vi "Camera_Widefield_old.vi"() -> ()   [LabVIEW 2014]
doc: "Allows the user to focus the camera on the sample"
uses:
  <vilib>/vision/Image Controls.llb/IMAQ Image.ctl
  <vilib>/userdefined/High Color/IMAQdx.ctl
  Widefield_globals.vi
  <vilib>/vision/NI_Vision_Development_Module.lvlib
  <vilib>/vision/driver/NI_Vision_Acquisition_Software.lvlib
  <resource>/objmgr/imaqdx.rc
panel:
  out "Exposure time (ms)":string
  out "Image Buffer":T1
  out "Waveform Graph":u32[](graph)
  in  "Snap":bool
  in  "Exit Focus Loop":bool
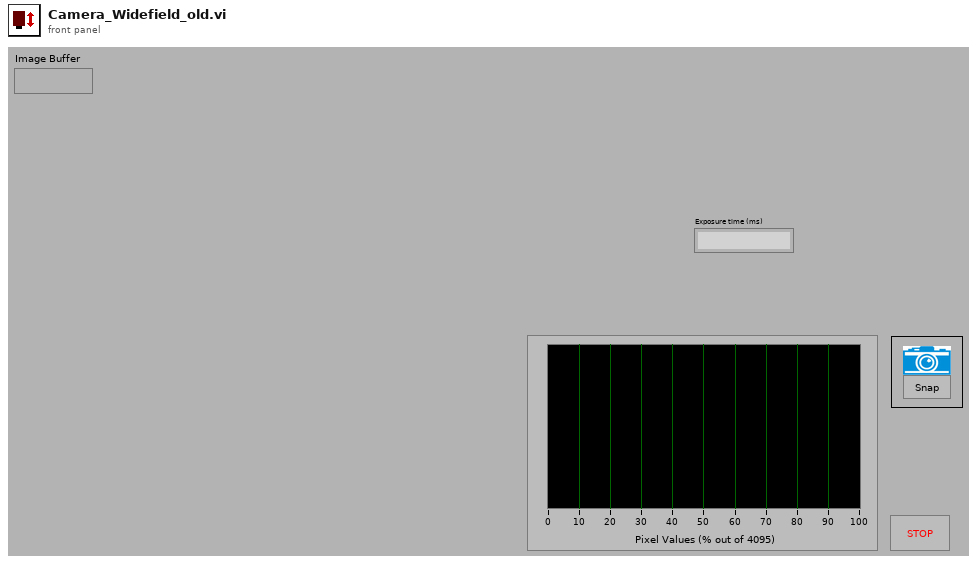
[diagram p1: front panel]
types:
  T1 = typedef "IMAQ Image.ctl" = refnum<image>
  T2 = typedef "IMAQdx.ctl" = refnum<k21>
  T3 = cluster{"histogram":u32[], "Minimal Value":sgl, "Maximal Value":sgl, "Starting Value":sgl, "Interval Width":sgl, "Mean Value":sgl, "Standard  Variation":sgl, "Area (pixels)":i32}
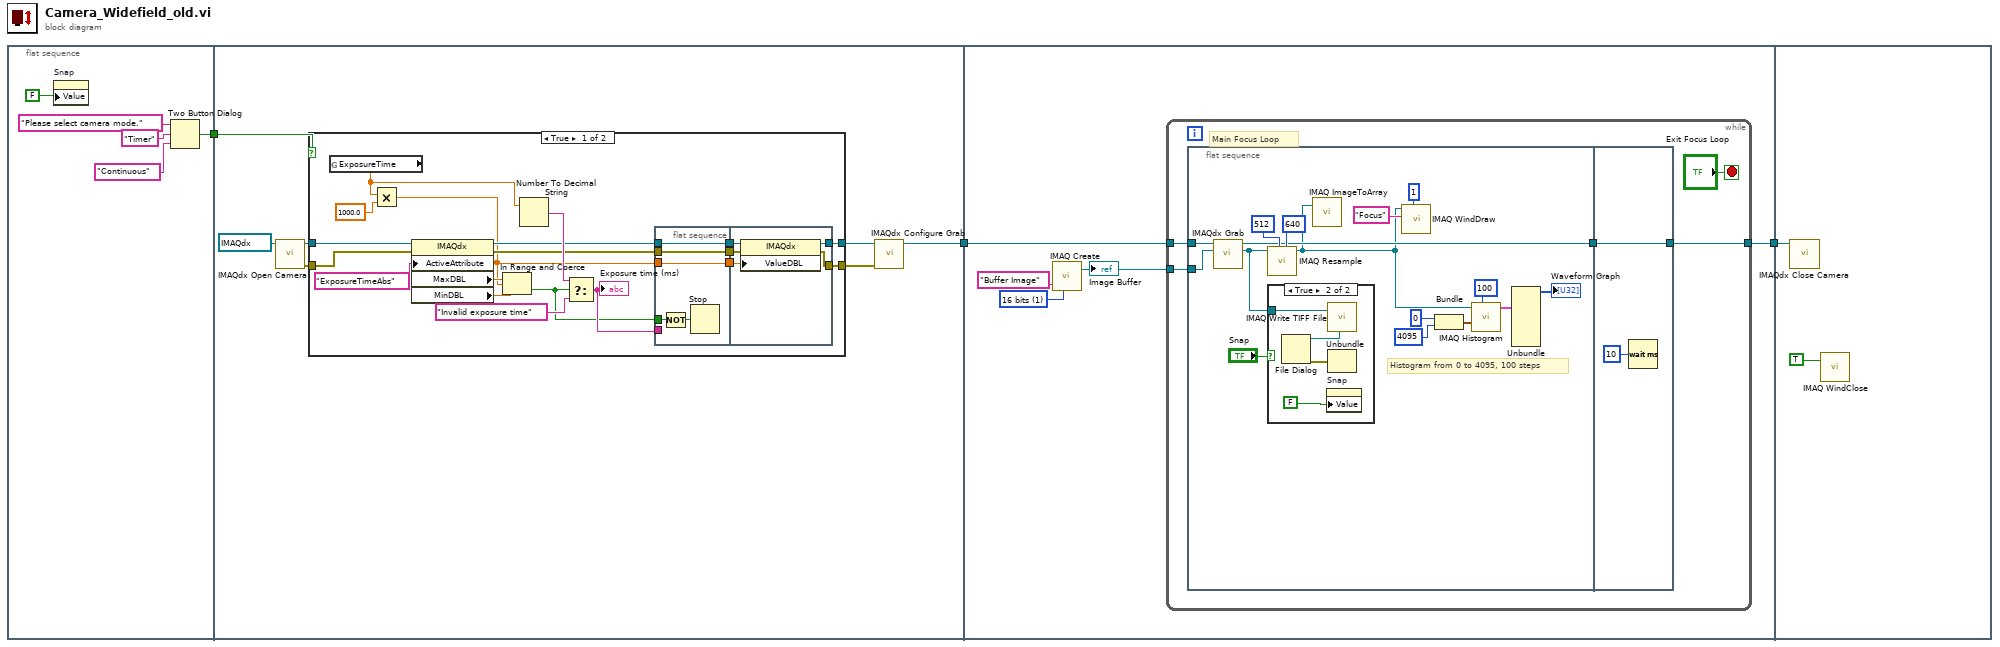
[diagram p0: block diagram]
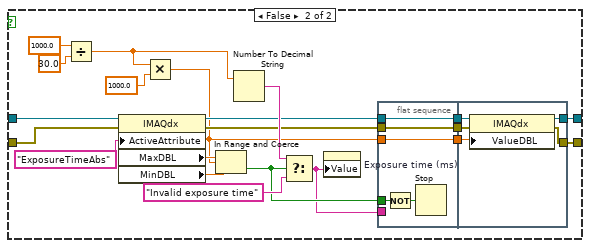
[diagram p2: hidden frame]
diagram:
  n1 = flat-sequence {
    tunnel: [w4] -> w3
    tunnel: w3 -> [w12]
    tunnel: [w9] -> w2
    tunnel: w2 -> [w77]
    tunnel: [w76] -> w1
    tunnel: w1 -> [w108]
    frame #0 {
      n2 = property on="Snap" class="Bool (strict)"("Value"=FALSE ("Snap!")) -> ()  [unwired: 2 in, 2 out]
      n3 = Two Button Dialog(message="Please select camera mode.", 1:"Continuous" ("F button name (\"Cancel\")"), 2:"Timer" ("T button name (\"OK\")")) -> (T button?=w4:bool)
    }
    frame #1 {
      n4 = call <vilib>:"IMAQdx Open Camera.vi"("Session In"=T2 "cam0") -> ("error out"=w13:errorcluster, "Session Out"=w14:T2)  [unwired: 2 in, 7 out]
      n5 = case shown="True" w12 {
        tunnel: [w18 w50] -> w15
        tunnel: w14 -> [w34 w65]
        tunnel: w13 -> [w32 w63]
        tunnel: [w19 w51] -> w10
        frame True {
          n6 = global read "Widefield_globals.vi" "ExposureTime"() -> (w16:dbl)
          n7 = Multiply(x=w16, y=1000.0) -> (x*y=w20:dbl)
          n8 = property class="IMAQdx"(reference=w34, error in=w32, "ActiveAttribute"="ExposureTimeAbs" ("Camera Attribute")) -> (reference out=w25:T2, error out=w24:errorcluster, "MaxDBL"=w31:dbl, "MinDBL"=w17:dbl)
          n9 = In Range and Coerce(upper limit=w31, x=w20, lower limit=w17) -> (In Range?=w26:bool)  [unwired: 1 out]
          n10 = Number To Decimal String(number=w16) -> (decimal integer string=w28:string)  [unwired: 1 out]
          n11 = Select(t=w28, s=w26, f="Invalid exposure time") -> (s? t:f=w27:string)
          "Exposure time (ms)" <- w27
          n12 = flat-sequence {
            tunnel: w27 -> [_]
            tunnel: w26 -> [w38]
            tunnel: w25 -> [w36]
            tunnel: w24 -> [w37]
            tunnel: [w37] -> w23
            tunnel: [w36] -> w22
            tunnel: [w35] -> w21
            tunnel: w20 -> [w35]
            tunnel: w23 -> [w43]
            tunnel: w22 -> [w44]
            tunnel: w21 -> [w42]
            tunnel: [w41] -> w19
            tunnel: [w40] -> w18
            frame #0 {
              n13 = Not(x=w38) -> (.not. x?=w39:bool)
              n14 = Stop(stop? (T)=w39) -> ()
            }
            frame #1 {
              n15 = property class="IMAQdx"(reference=w44, error in=w43, "ValueDBL"=w42) -> (reference out=w41:T2, error out=w40:errorcluster)
            }
          }
        }
        frame False {
          n16 = Divide(x=1000.0 ("y"), y=30.0) -> (x/y=w46:dbl)
          n17 = property class="IMAQdx"(reference=w65, error in=w63, "ActiveAttribute"="ExposureTimeAbs" ("Camera Attribute")) -> (reference out=w57:T2, error out=w56:errorcluster, "MaxDBL"=w62:dbl, "MinDBL"=w49:dbl)
          n18 = Multiply(x=w46, y=1000.0) -> (x*y=w52:dbl)
          n19 = In Range and Coerce(upper limit=w62, x=w52, lower limit=w49) -> (In Range?=w58:bool)  [unwired: 1 out]
          n20 = Number To Decimal String(number=w46) -> (decimal integer string=w59:string)  [unwired: 1 out]
          n21 = Select(t=w59, s=w58, f="Invalid exposure time") -> (s? t:f=w45:string)
          n22 = property on="Exposure time (ms)" class="Str"("Value"=w45) -> ()  [unwired: 2 in, 2 out]
          n23 = flat-sequence {
            tunnel: w45 -> [_]
            tunnel: w58 -> [w69]
            tunnel: w57 -> [w67]
            tunnel: w56 -> [w68]
            tunnel: [w68] -> w55
            tunnel: [w67] -> w54
            tunnel: [w66] -> w53
            tunnel: w52 -> [w66]
            tunnel: w55 -> [w74]
            tunnel: w54 -> [w75]
            tunnel: w53 -> [w73]
            tunnel: [w72] -> w51
            tunnel: [w71] -> w50
            frame #0 {
              n24 = Not(x=w69) -> (.not. x?=w70:bool)
              n25 = Stop(stop? (T)=w70) -> ()
            }
            frame #1 {
              n26 = property class="IMAQdx"(reference=w75, error in=w74, "ValueDBL"=w73) -> (reference out=w72:T2, error out=w71:errorcluster)
            }
          }
        }
      }
      n27 = call <vilib>:"IMAQdx Configure Grab.vi"("error in"=w15, "Session In"=w10) -> ("Session Out"=w9:T2)  [unwired: 9 out]
    }
    frame #2 {
      w79 = u32 1 items=["8 bits", "16 bits", "Float", "Complex", "RGB", "HSL"] ("Image Type")
      n28 = call "IMAQ Create"("Image Name"="Buffer Image", "Image Type"=w79) -> ("New Image"=w78:T1)  [unwired: 2 in, 2 out]
      "Image Buffer" <- w78
      n29 = while {
        tunnel: w78 -> [w84]
        tunnel: w77 -> [w81]
        tunnel: [w83] -> w76
        stop <- "Exit Focus Loop" stop-if-true
        # "Main Focus Loop"
        n30 = flat-sequence {
          tunnel: w84 -> [w89]
          tunnel: [w88] -> w82
          tunnel: w81 -> [w87]
          tunnel: [w106] -> w83
          tunnel: w82 -> [w106]
          frame #0 {
            # "Histogram from 0 to 4095, 100 steps"
            n31 = call <vilib>:"IMAQdx Grab.vi"("Image In"=w89, "Session In"=w87) -> ("Image Out"=w90:T1, "Session Out"=w88:T2)  [unwired: 2 in, 6 out]
            n32 = call "IMAQ Resample"("X Resolution"=640, "Y Resolution"=512, "Image Src"=w90) -> ("Image Dst Out"=w86:T1)  [unwired: 4 in, 4 out]
            n33 = case shown="True" "Snap" {
              tunnel: w90 -> [_ w104]
              frame False {
              }
              frame True {
                n34 = File Dialog() -> (0:w103:errorcluster, 3:w105:path)  [unwired: 1 in, 8 out]
                n35 = property on="Snap" class="Bool (strict)"("Value"=FALSE ("Snap!")) -> ()  [unwired: 2 in, 2 out]
                n36 = call "IMAQ Write TIFF File"("File Path"=w105, "Image"=w104) -> ()  [unwired: 3 in, 4 out]
                n37 = Unbundle(w103) -> ()  [unwired: 3 out]
              }
            }
            n38 = call "IMAQ ImageToArray"("Image"=w86) -> ()  [unwired: 2 in, 6 out]
            n39 = call "IMAQ WindDraw"("Window Number (0...15)"=1, "Title"="Focus", "Image"=w86) -> ()  [unwired: 3 in, 6 out]
            n40 = Bundle(0, 4095) -> (w91:cluster{i32, i32})  [unwired: 1 out]
            n41 = call "IMAQ Histogram"("Number of Classes"=100, "Interval Range"=w91, "Image"=w86) -> ("Histogram Report"=w96:T3)  [unwired: 2 in, 6 out]
            n42 = Unbundle(w96) -> ("histogram"=→"Waveform Graph":u32[])  [unwired: 7 out]
          }
          frame #1 {
            n43 = Wait (ms)(milliseconds to wait=u32 10) -> ()  [unwired: 1 out]
          }
        }
      }
    }
    frame #3 {
      n44 = call <vilib>:"IMAQdx Close Camera.vi"("Session In"=w108) -> ()  [unwired: 1 in, 10 out]
      n45 = call "IMAQ WindClose"("Close All Windows (False)"=TRUE) -> ()  [unwired: 2 in, 4 out]
    }
  }
